vi "总磷总氮测量数据储存.vi"   [LabVIEW 2016, in "斯坦道总氮.lvlib"]
types:
  T1 = enum16{"水样测试", "标样核查", "跨度核查", "零点核查", "加标回收", "空白测试", "平行样"}
  T2 = cluster{"时间标识":timestamp, "测量模式":enum16{"维护数据", "水样测试", "标样核查", "零点核查", "跨度核查", "空白测试", "平行样测试", "加标回收", "空白校准", "标样校准", "初始化（清洗）"}, "数据标记表":string, "监测值":sgl, "单位":u16, "数据标识":string, "因子编码":u32, "标样参考值":sgl, "F0":sgl, "F1":sgl, "F2":sgl, "F3":sgl, "F4":sgl, "F5":sgl, "F6":sgl, "F7":sgl, "X":sgl, "温度":sgl, "湿度":sgl, "量程标识":string, "SN":string}
  T3 = enum16{"维护数据", "水样测试", "标样核查", "零点核查", "跨度核查", "空白测试", "平行样测试", "加标回收", "空白校准", "标样校准", "初始化（清洗）"}
  T4 = cluster{"系统时间":timestamp, "工作状态":enum16{"空闲", "水样测试", "标样核查", "零点核查", "跨度核查", "空白测试", "平行样测试", "加标回收", "空白校准", "标样校准", "初始化（清洗）"}, "测量模式":enum16{"待机", "连续模式", "周期模式", "定点模式", "受控模式", "手动模式"}, "告警代码":u16, "故障代码":u16, "日志代码":u16, "软件版本":u16, "F0":sgl, "F1":sgl, "F2":sgl, "F3":sgl, "T":sgl, "H":sgl, "id":u16, "flowid":u16, "量程":u16, "总磷控温温度1":sgl, "营养盐控温温度2":sgl, "ADC":sgl}
  T5 = cluster{"运行模式":enum16{"维护模式", "常规模式", "应急模式", "质控模式"}, "质控频次":enum16{"关闭", "每天", "星期一", "星期二", "星期三", "星期四", "星期五", "星期六", "星期日"}, "空白核查时间":u16, "跨度核查时间":u16, "24H周期设置":bool[]}
  T6 = enum16{"空闲", "水样测试", "标样核查", "零点核查", "跨度核查", "空白测试", "平行样测试", "加标回收", "空白校准", "标样校准", "初始化（清洗）"}
  T7 = cluster{"因子编码":u32, "单位":u16, "标样参考值":sgl, "水样数据时间":timestamp, "水样实测值":sgl, "水样数据标识":string, "标样数据时间":timestamp, "标样实测值":sgl, "标样数据标识":string, "空白数据时间":timestamp, "空白实测值":sgl, "空白数据标识":string, "零点核查数据时间":timestamp, "零点核查实测值":sgl, "零点核查数据标识":string, "跨度核查数据时间":timestamp, "跨度核查实测值":sgl, "跨度核查数据标识":string, "加标回收数据时间":timestamp, "加标回收实测值":sgl, "加标回收数据标识":string, "平行样数据时间":timestamp, "平行样实测值":sgl, "平行样数据标识":string, "F0":sgl, "F1":sgl, "F2":sgl, "F3":sgl, "F4":sgl, "F5":sgl, "F6":sgl, "F7":sgl, "温度":sgl, "湿度":sgl, "X值":sgl, "fidrange":u16}
  T8 = cluster{"总磷跨度值":dbl, "总磷零点标准液浓度":dbl, "总磷跨度标准液浓度":dbl, "总磷标准液标准浓度":dbl, "总氮跨度值":dbl, "总氮零点标准液浓度":dbl, "总氮跨度标准液浓度":dbl, "总氮标准液标准浓度":dbl, "COD跨度值":dbl, "COD零点标准液浓度":dbl, "COD跨度标准液浓度":dbl, "COD标准液标准浓度":dbl, "氨氮跨度值":dbl, "氨氮零点标准液浓度":dbl, "氨氮跨度标准液浓度":dbl, "氨氮标准液标准浓度":dbl}
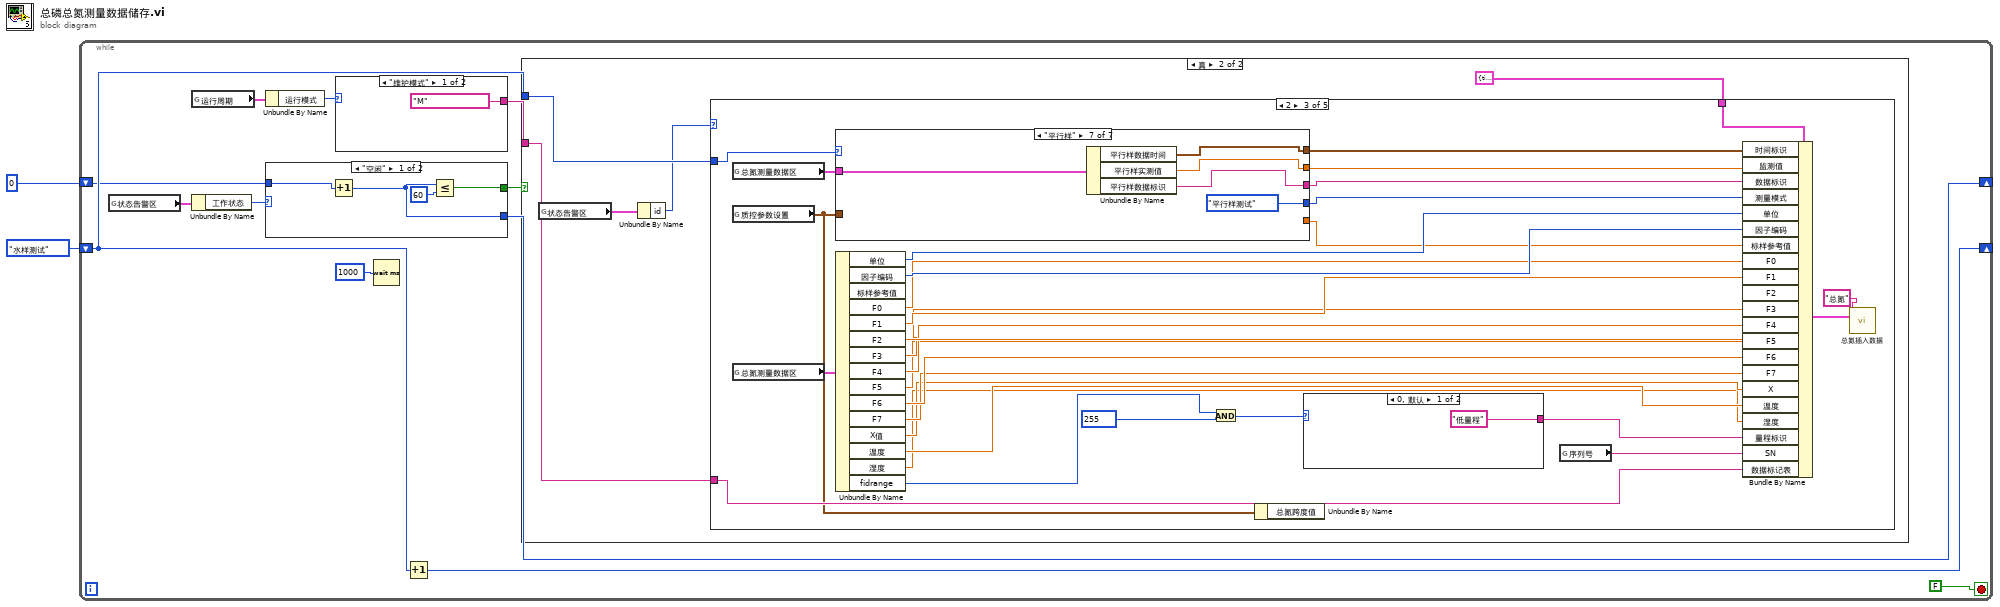
[diagram p0: block diagram]
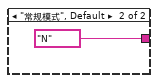
[diagram p3: hidden frame]
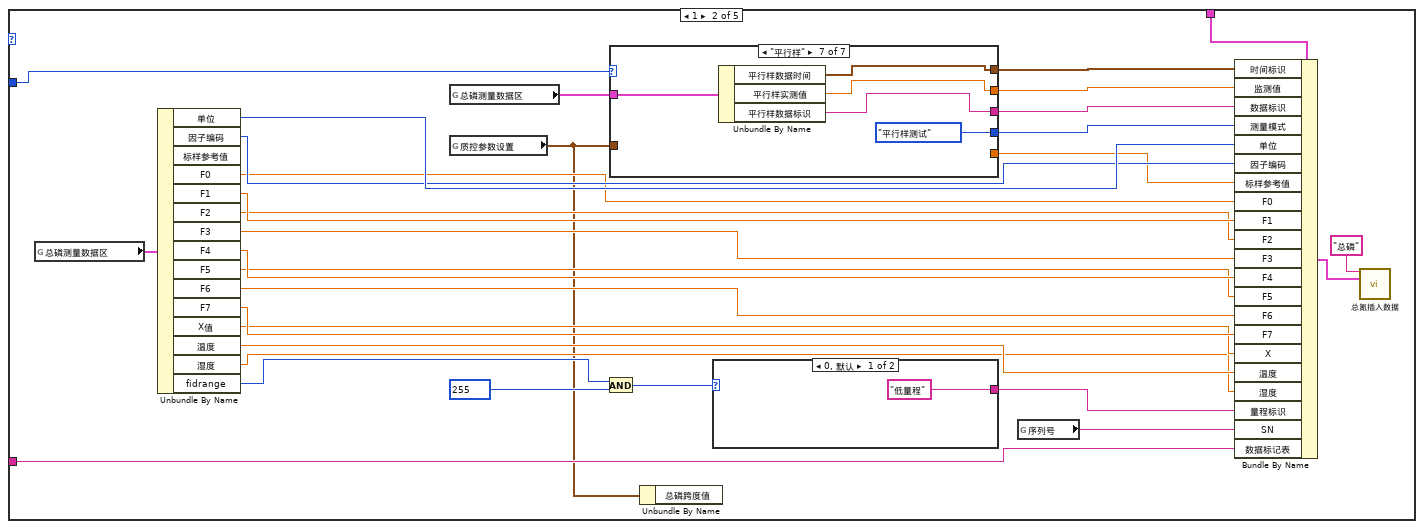
[diagram p6: hidden frame]
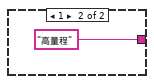
[diagram p7: hidden frame]
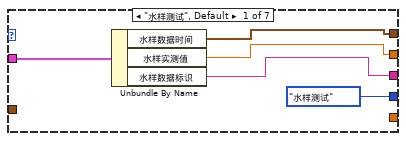
[diagram p8: hidden frame]
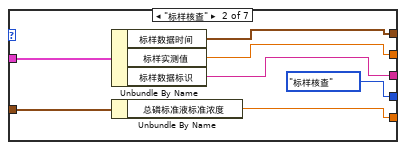
[diagram p9: hidden frame]
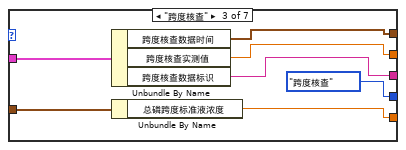
[diagram p10: hidden frame]
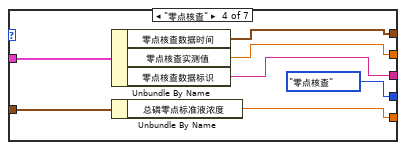
[diagram p11: hidden frame]
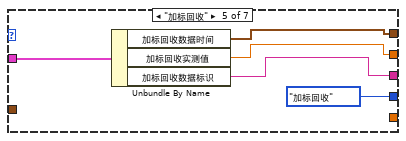
[diagram p12: hidden frame]
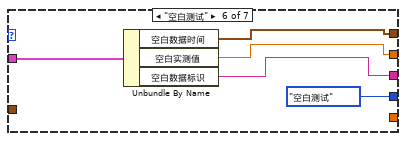
[diagram p13: hidden frame]
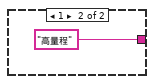
[diagram p14: hidden frame]
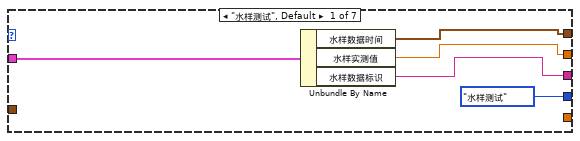
[diagram p15: hidden frame]
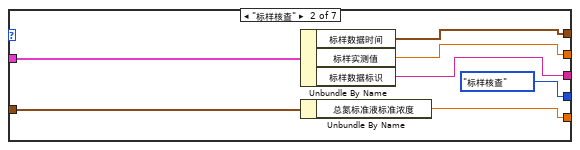
[diagram p16: hidden frame]
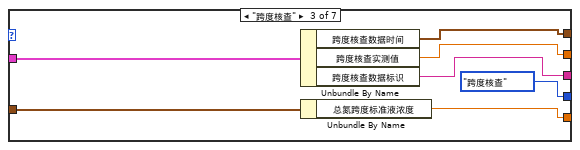
[diagram p17: hidden frame]
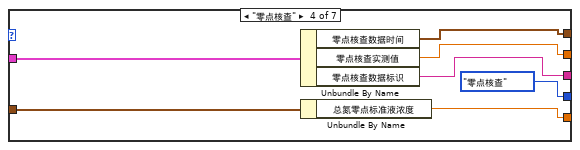
[diagram p18: hidden frame]
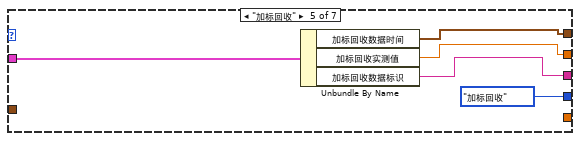
[diagram p19: hidden frame]
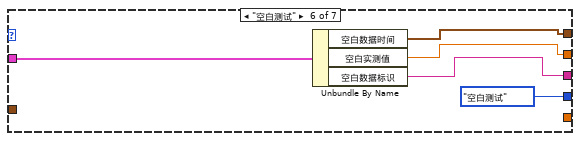
[diagram p20: hidden frame]
diagram:
  n1 = while {
    shift-right: [w12] -> _
    shift-left: T1."水样测试" ("测量模式") -> [w11]
    shift-right: [w5] -> _
    shift-left: u32 0 ("等待时间（毫秒）") -> [w6]
    stop <- FALSE stop-if-true
    n2 = global read "VAR总磷总氮全局变量.vi" "状态告警区"() -> (w8:T4)
    n3 = global read "总磷总氮断电保存全局变量.vi" "运行周期"() -> (w10:T5)
    n4 = Unbundle By Name(w8) -> ("工作状态"=w7:T6)
    n5 = Unbundle By Name(w10) -> ("运行模式"=w9:enum16{"维护模式", "常规模式", "应急模式", "质控模式"})
    n6 = case shown="\"空闲\"" w7 {
      tunnel: w6 -> [w18 _]
      tunnel: [w17 _] -> w5
      tunnel: [w15 _] -> w4
      frame "空闲" {
        n7 = Increment(x=w18) -> (x+1=w17:u32)
        n8 = Less Or Equal?(x=w17, y=u32 60) -> (x <= y?=w15:bool)
      }
      frame "水样测试", Default {
      }
    }
    n9 = case shown="\"维护模式\"" w9 {
      tunnel: ["M" ("数据标记表") "N" ("数据标记表")] -> w13
      frame "维护模式" {
      }
      frame "常规模式", Default {
      }
    }
    n10 = Wait (ms)(milliseconds to wait=u32 1000 ("等待时间（毫秒）")) -> ()  [unwired: 1 out]
    n11 = Increment(x=w11) -> (x+1=w12:T1)
    n12 = case shown="真" w4 {
      tunnel: w13 -> [_ w25]
      tunnel: w11 -> [_ w24]
      frame False {
      }
      frame True {
        n13 = global read "VAR总磷总氮全局变量.vi" "状态告警区"() -> (w23:T4)
        n14 = Unbundle By Name(w23) -> ("id"=w22:u16)
        n15 = case shown="2" w22 {
          tunnel: w25 -> [_ w31 w105 w179 w253]
          tunnel: w24 -> [_ w38 w116 w190 w264]
          tunnel: T2 {"时间标识"=timestamp(0 s since 1904-01-01), "测量模式"=enum."水样测试", "数据标记表"="N", "监测值"=0.0, "单位"=0, "数据标识"="", "因子编码"=0, "标样参考值"=0.0, "F0"=0.0, "F1"=0.0, "F2"=0.0, "F3"=0.0, "F4"=0.0, "F5"=0.0, "F6"=0.0, "F7"=0.0, "X"=0.0, "温度"=0.0, "湿度"=0.0, "量程标识"="", "SN"=""} ("data") -> [_ w29 w103 w177 w251]
          frame Default {
          }
          frame 1 {
            n16 = global read "VAR总磷总氮全局变量.vi" "总磷测量数据区"() -> (w42:T7)
            n17 = Unbundle By Name(w42) -> ("单位"=w55:u16, "因子编码"=w54:u32, "F0"=w53:sgl, "F1"=w52:sgl, "F2"=w51:sgl, "F3"=w50:sgl, "F4"=w49:sgl, "F5"=w48:sgl, "F6"=w47:sgl, "F7"=w46:sgl, "X值"=w45:sgl, "温度"=w44:sgl, "湿度"=w43:sgl, "fidrange"=w36:u16)  [unwired: 1 out]
            n18 = global read "VAR总磷总氮全局变量.vi" "总磷测量数据区"() -> (w56:T7)
            n19 = global read "总磷总氮断电保存全局变量.vi" "质控参数设置"() -> (w28:T8)
            n20 = And(x=w36, y=u16 255) -> (x .and. y?=w34:u16)
            n21 = case shown="\"平行样\"" w38 {
              tunnel: w56 -> [w63 w70 w77 w84 w89 w94 w99]
              tunnel: [w62 w69 w76 w83 w88 w93 w98] -> w39
              tunnel: [w61 w68 w75 w82 w87 w92 w97] -> w40
              tunnel: [w60 w67 w74 w81 w86 w91 w96] -> w41
              tunnel: [T3."水样测试" ("测量模式") T3."标样核查" ("测量模式") T3."跨度核查" ("测量模式") T3."零点核查" ("测量模式") T3."加标回收" ("测量模式") T3."空白测试" ("测量模式") T3."平行样测试" ("测量模式")] -> w30
              tunnel: w28 -> [_ w65 w72 w79 _ _ _]
              tunnel: [_ w64 w71 w78 _ _ _] -> w37
              frame "水样测试", Default {
                n22 = Unbundle By Name(w63) -> ("水样数据时间"=w62:timestamp, "水样实测值"=w61:sgl, "水样数据标识"=w60:string)
              }
              frame "标样核查" {
                n23 = Unbundle By Name(w70) -> ("标样数据时间"=w69:timestamp, "标样实测值"=w68:sgl, "标样数据标识"=w67:string)
                n24 = Unbundle By Name(w65) -> ("总磷标准液标准浓度"=w64:dbl)
              }
              frame "跨度核查" {
                n25 = Unbundle By Name(w77) -> ("跨度核查数据时间"=w76:timestamp, "跨度核查实测值"=w75:sgl, "跨度核查数据标识"=w74:string)
                n26 = Unbundle By Name(w72) -> ("总磷跨度标准液浓度"=w71:dbl)
              }
              frame "零点核查" {
                n27 = Unbundle By Name(w84) -> ("零点核查数据时间"=w83:timestamp, "零点核查实测值"=w82:sgl, "零点核查数据标识"=w81:string)
                n28 = Unbundle By Name(w79) -> ("总磷零点标准液浓度"=w78:dbl)
              }
              frame "加标回收" {
                n29 = Unbundle By Name(w89) -> ("加标回收数据时间"=w88:timestamp, "加标回收实测值"=w87:sgl, "加标回收数据标识"=w86:string)
              }
              frame "空白测试" {
                n30 = Unbundle By Name(w94) -> ("空白数据时间"=w93:timestamp, "空白实测值"=w92:sgl, "空白数据标识"=w91:string)
              }
              frame "平行样" {
                n31 = Unbundle By Name(w99) -> ("平行样数据时间"=w98:timestamp, "平行样实测值"=w97:sgl, "平行样数据标识"=w96:string)
              }
            }
            n32 = Unbundle By Name(w28) -> ()  [unwired: 1 out]
            n33 = case shown="0, 默认" w34 {
              tunnel: ["低量程" ("格式字符串") "高量程" ("格式字符串")] -> w33
              frame 0, Default {
              }
              frame 1 {
              }
            }
            n34 = global read "VAR总磷总氮全局变量.vi" "序列号"() -> (w32:string)
            n35 = Bundle By Name(cluster=w29, "时间标识"=w39, "监测值"=w40, "数据标识"=w41, "测量模式"=w30, "单位"=w55, "因子编码"=w54, "标样参考值"=w37, "F0"=w53, "F1"=w52, "F2"=w51, "F3"=w50, "F4"=w49, "F5"=w48, "F6"=w47, "F7"=w46, "X"=w45, "温度"=w44, "湿度"=w43, "量程标识"=w33, "SN"=w32, "数据标记表"=w31) -> (w26:T2)
            n36 = call "总氮插入数据.vi"("table"="总磷", "data"=w26) -> ()  [unwired: 13 in, 1 out]
          }
          frame 2 {
            n37 = global read "VAR总磷总氮全局变量.vi" "总氮测量数据区"() -> (w115:T7)
            n38 = global read "总磷总氮断电保存全局变量.vi" "质控参数设置"() -> (w102:T8)
            n39 = global read "VAR总磷总氮全局变量.vi" "总氮测量数据区"() -> (w130:T7)
            n40 = case shown="\"平行样\"" w116 {
              tunnel: w115 -> [w137 w144 w151 w158 w163 w168 w173]
              tunnel: [w136 w143 w150 w157 w162 w167 w172] -> w114
              tunnel: [w135 w142 w149 w156 w161 w166 w171] -> w113
              tunnel: [w134 w141 w148 w155 w160 w165 w170] -> w112
              tunnel: [T3."水样测试" ("测量模式") T3."标样核查" ("测量模式") T3."跨度核查" ("测量模式") T3."零点核查" ("测量模式") T3."加标回收" ("测量模式") T3."空白测试" ("测量模式") T3."平行样测试" ("测量模式")] -> w104
              tunnel: w102 -> [_ w139 w146 w153 _ _ _]
              tunnel: [_ w138 w145 w152 _ _ _] -> w111
              frame "水样测试", Default {
                n41 = Unbundle By Name(w137) -> ("水样数据时间"=w136:timestamp, "水样实测值"=w135:sgl, "水样数据标识"=w134:string)
              }
              frame "标样核查" {
                n42 = Unbundle By Name(w144) -> ("标样数据时间"=w143:timestamp, "标样实测值"=w142:sgl, "标样数据标识"=w141:string)
                n43 = Unbundle By Name(w139) -> ("总氮标准液标准浓度"=w138:dbl)
              }
              frame "跨度核查" {
                n44 = Unbundle By Name(w151) -> ("跨度核查数据时间"=w150:timestamp, "跨度核查实测值"=w149:sgl, "跨度核查数据标识"=w148:string)
                n45 = Unbundle By Name(w146) -> ("总氮跨度标准液浓度"=w145:dbl)
              }
              frame "零点核查" {
                n46 = Unbundle By Name(w158) -> ("零点核查数据时间"=w157:timestamp, "零点核查实测值"=w156:sgl, "零点核查数据标识"=w155:string)
                n47 = Unbundle By Name(w153) -> ("总氮零点标准液浓度"=w152:dbl)
              }
              frame "加标回收" {
                n48 = Unbundle By Name(w163) -> ("加标回收数据时间"=w162:timestamp, "加标回收实测值"=w161:sgl, "加标回收数据标识"=w160:string)
              }
              frame "空白测试" {
                n49 = Unbundle By Name(w168) -> ("空白数据时间"=w167:timestamp, "空白实测值"=w166:sgl, "空白数据标识"=w165:string)
              }
              frame "平行样" {
                n50 = Unbundle By Name(w173) -> ("平行样数据时间"=w172:timestamp, "平行样实测值"=w171:sgl, "平行样数据标识"=w170:string)
              }
            }
            n51 = Unbundle By Name(w130) -> ("单位"=w129:u16, "因子编码"=w128:u32, "F0"=w127:sgl, "F1"=w126:sgl, "F2"=w125:sgl, "F3"=w124:sgl, "F4"=w123:sgl, "F5"=w122:sgl, "F6"=w121:sgl, "F7"=w120:sgl, "X值"=w119:sgl, "温度"=w118:sgl, "湿度"=w117:sgl, "fidrange"=w108:u16)  [unwired: 1 out]
            n52 = And(x=w108, y=u16 255) -> (x .and. y?=w109:u16)
            n53 = Unbundle By Name(w102) -> ()  [unwired: 1 out]
            n54 = case shown="0, 默认" w109 {
              tunnel: ["低量程" ("格式字符串") "高量程" ("格式字符串")] -> w107
              frame 0, Default {
              }
              frame 1 {
              }
            }
            n55 = global read "VAR总磷总氮全局变量.vi" "序列号"() -> (w106:string)
            n56 = Bundle By Name(cluster=w103, "时间标识"=w114, "监测值"=w113, "数据标识"=w112, "测量模式"=w104, "单位"=w129, "因子编码"=w128, "标样参考值"=w111, "F0"=w127, "F1"=w126, "F2"=w125, "F3"=w124, "F4"=w123, "F5"=w122, "F6"=w121, "F7"=w120, "X"=w119, "温度"=w118, "湿度"=w117, "量程标识"=w107, "SN"=w106, "数据标记表"=w105) -> (w100:T2)
            n57 = call "总氮插入数据.vi"("table"="总氮", "data"=w100) -> ()  [unwired: 13 in, 1 out]
          }
          frame 3 {
            n58 = global read "VAR总磷总氮全局变量.vi" "氨氮测量数据区"() -> (w189:T7)
            n59 = global read "总磷总氮断电保存全局变量.vi" "质控参数设置"() -> (w176:T8)
            n60 = global read "VAR总磷总氮全局变量.vi" "氨氮测量数据区"() -> (w204:T7)
            n61 = case shown="\"平行样\"" w190 {
              tunnel: w189 -> [w211 w218 w225 w232 w237 w242 w247]
              tunnel: [w210 w217 w224 w231 w236 w241 w246] -> w188
              tunnel: [w209 w216 w223 w230 w235 w240 w245] -> w187
              tunnel: [w208 w215 w222 w229 w234 w239 w244] -> w186
              tunnel: [T3."水样测试" ("测量模式") T3."标样核查" ("测量模式") T3."跨度核查" ("测量模式") T3."零点核查" ("测量模式") T3."加标回收" ("测量模式") T3."空白测试" ("测量模式") T3."平行样测试" ("测量模式")] -> w178
              tunnel: w176 -> [_ w213 w220 w227 _ _ _]
              tunnel: [_ w212 w219 w226 _ _ _] -> w185
              frame "水样测试", Default {
                n62 = Unbundle By Name(w211) -> ("水样数据时间"=w210:timestamp, "水样实测值"=w209:sgl, "水样数据标识"=w208:string)
              }
              frame "标样核查" {
                n63 = Unbundle By Name(w218) -> ("标样数据时间"=w217:timestamp, "标样实测值"=w216:sgl, "标样数据标识"=w215:string)
                n64 = Unbundle By Name(w213) -> ("氨氮标准液标准浓度"=w212:dbl)
              }
              frame "跨度核查" {
                n65 = Unbundle By Name(w225) -> ("跨度核查数据时间"=w224:timestamp, "跨度核查实测值"=w223:sgl, "跨度核查数据标识"=w222:string)
                n66 = Unbundle By Name(w220) -> ("氨氮跨度标准液浓度"=w219:dbl)
              }
              frame "零点核查" {
                n67 = Unbundle By Name(w232) -> ("零点核查数据时间"=w231:timestamp, "零点核查实测值"=w230:sgl, "零点核查数据标识"=w229:string)
                n68 = Unbundle By Name(w227) -> ("氨氮零点标准液浓度"=w226:dbl)
              }
              frame "加标回收" {
                n69 = Unbundle By Name(w237) -> ("加标回收数据时间"=w236:timestamp, "加标回收实测值"=w235:sgl, "加标回收数据标识"=w234:string)
              }
              frame "空白测试" {
                n70 = Unbundle By Name(w242) -> ("空白数据时间"=w241:timestamp, "空白实测值"=w240:sgl, "空白数据标识"=w239:string)
              }
              frame "平行样" {
                n71 = Unbundle By Name(w247) -> ("平行样数据时间"=w246:timestamp, "平行样实测值"=w245:sgl, "平行样数据标识"=w244:string)
              }
            }
            n72 = Unbundle By Name(w204) -> ("单位"=w203:u16, "因子编码"=w202:u32, "F0"=w201:sgl, "F1"=w200:sgl, "F2"=w199:sgl, "F3"=w198:sgl, "F4"=w197:sgl, "F5"=w196:sgl, "F6"=w195:sgl, "F7"=w194:sgl, "X值"=w193:sgl, "温度"=w192:sgl, "湿度"=w191:sgl, "fidrange"=w182:u16)  [unwired: 1 out]
            n73 = And(x=w182, y=u16 255) -> (x .and. y?=w183:u16)
            n74 = Unbundle By Name(w176) -> ()  [unwired: 1 out]
            n75 = case shown="0, 默认" w183 {
              tunnel: ["低量程" ("格式字符串") "高量程" ("格式字符串")] -> w181
              frame 0, Default {
              }
              frame 1 {
              }
            }
            n76 = global read "VAR总磷总氮全局变量.vi" "序列号"() -> (w180:string)
            n77 = Bundle By Name(cluster=w177, "时间标识"=w188, "监测值"=w187, "数据标识"=w186, "测量模式"=w178, "单位"=w203, "因子编码"=w202, "标样参考值"=w185, "F0"=w201, "F1"=w200, "F2"=w199, "F3"=w198, "F4"=w197, "F5"=w196, "F6"=w195, "F7"=w194, "X"=w193, "温度"=w192, "湿度"=w191, "量程标识"=w181, "SN"=w180, "数据标记表"=w179) -> (w174:T2)
            n78 = call "总氮插入数据.vi"("table"="氨氮", "data"=w174) -> ()  [unwired: 13 in, 1 out]
          }
          frame 22 {
            n79 = global read "VAR总磷总氮全局变量.vi" "COD测量数据区"() -> (w263:T7)
            n80 = global read "VAR总磷总氮全局变量.vi" "COD测量数据区"() -> (w278:T7)
            n81 = global read "总磷总氮断电保存全局变量.vi" "质控参数设置"() -> (w250:T8)
            n82 = case shown="\"平行样\"" w264 {
              tunnel: w263 -> [w285 w292 w299 w306 w311 w316 w321]
              tunnel: [w284 w291 w298 w305 w310 w315 w320] -> w262
              tunnel: [w283 w290 w297 w304 w309 w314 w319] -> w261
              tunnel: [w282 w289 w296 w303 w308 w313 w318] -> w260
              tunnel: [T3."水样测试" ("测量模式") T3."标样核查" ("测量模式") T3."跨度核查" ("测量模式") T3."零点核查" ("测量模式") T3."加标回收" ("测量模式") T3."空白测试" ("测量模式") T3."平行样测试" ("测量模式")] -> w252
              tunnel: w250 -> [_ w287 w294 w301 _ _ _]
              tunnel: [_ w286 w293 w300 _ _ _] -> w259
              frame "水样测试", Default {
                n83 = Unbundle By Name(w285) -> ("水样数据时间"=w284:timestamp, "水样实测值"=w283:sgl, "水样数据标识"=w282:string)
              }
              frame "标样核查" {
                n84 = Unbundle By Name(w287) -> ("COD标准液标准浓度"=w286:dbl)
                n85 = Unbundle By Name(w292) -> ("标样数据时间"=w291:timestamp, "标样实测值"=w290:sgl, "标样数据标识"=w289:string)
              }
              frame "跨度核查" {
                n86 = Unbundle By Name(w294) -> ("COD跨度标准液浓度"=w293:dbl)
                n87 = Unbundle By Name(w299) -> ("跨度核查数据时间"=w298:timestamp, "跨度核查实测值"=w297:sgl, "跨度核查数据标识"=w296:string)
              }
              frame "零点核查" {
                n88 = Unbundle By Name(w301) -> ("COD零点标准液浓度"=w300:dbl)
                n89 = Unbundle By Name(w306) -> ("零点核查数据时间"=w305:timestamp, "零点核查实测值"=w304:sgl, "零点核查数据标识"=w303:string)
              }
              frame "加标回收" {
                n90 = Unbundle By Name(w311) -> ("加标回收数据时间"=w310:timestamp, "加标回收实测值"=w309:sgl, "加标回收数据标识"=w308:string)
              }
              frame "空白测试" {
                n91 = Unbundle By Name(w316) -> ("空白数据时间"=w315:timestamp, "空白实测值"=w314:sgl, "空白数据标识"=w313:string)
              }
              frame "平行样" {
                n92 = Unbundle By Name(w321) -> ("平行样数据时间"=w320:timestamp, "平行样实测值"=w319:sgl, "平行样数据标识"=w318:string)
              }
            }
            n93 = Unbundle By Name(w278) -> ("单位"=w277:u16, "因子编码"=w276:u32, "F0"=w275:sgl, "F1"=w274:sgl, "F2"=w273:sgl, "F3"=w272:sgl, "F4"=w271:sgl, "F5"=w270:sgl, "F6"=w269:sgl, "F7"=w268:sgl, "X值"=w267:sgl, "温度"=w266:sgl, "湿度"=w265:sgl, "fidrange"=w256:u16)  [unwired: 1 out]
            n94 = Unbundle By Name(w250) -> ()  [unwired: 1 out]
            n95 = And(x=w256, y=u16 255) -> (x .and. y?=w257:u16)
            n96 = case shown="0, 默认" w257 {
              tunnel: ["低量程" ("格式字符串") "高量程" ("格式字符串")] -> w255
              frame 0, Default {
              }
              frame 1 {
              }
            }
            n97 = global read "VAR总磷总氮全局变量.vi" "序列号"() -> (w254:string)
            n98 = Bundle By Name(cluster=w251, "时间标识"=w262, "监测值"=w261, "数据标识"=w260, "测量模式"=w252, "单位"=w277, "因子编码"=w276, "标样参考值"=w259, "F0"=w275, "F1"=w274, "F2"=w273, "F3"=w272, "F4"=w271, "F5"=w270, "F6"=w269, "F7"=w268, "X"=w267, "温度"=w266, "湿度"=w265, "量程标识"=w255, "SN"=w254, "数据标记表"=w253) -> (w248:T2)
            n99 = call "总氮插入数据.vi"("table"="COD", "data"=w248) -> ()  [unwired: 13 in, 1 out]
          }
        }
      }
    }
  }
